vi "Get Valid Properties.vi"(8 "error in (no error)":errorcluster, 11 "SAM in":refnum<class "SAM.lvclass">) -> (0 "error out":errorcluster, 2 "Properties":string[](array[string]), 3 "SAM out":refnum<class "SAM.lvclass">)   [LabVIEW 2020, in "SAM.lvclass"]
uses:
  SAM.lvclass
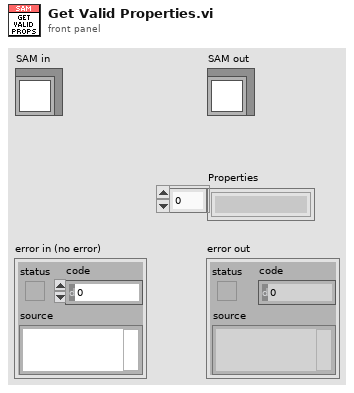
[diagram p1: front panel]
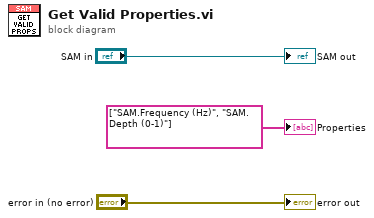
[diagram p0: block diagram]
diagram:
  "error out" <- "error in (no error)"
  "SAM out" <- "SAM in"
  "Properties" <- string[] ["SAM.Frequency (Hz)", "SAM.Depth (0-1)"] ("Properties")
